vi "CRYResonance Fit.vi"(6 "Y data":dbl=1.0, 7 "Y ref":dbl=1.0, 8 "Algorithm (0)":i32 min=0 max=2 step=1, 11 "Input":cluster{"Freq":dbl, "Magn":dbl}[](array[cluster]) {"Magn" format="%.4f"; "Freq" format="%.2f"}) -> (0 "error":i32, 1 "Q":dbl format="%.2f", 2 "Magn":dbl format="%.2f", 3 "Freq":dbl format="%.2f", 4 "Output":cluster{"FStart":dbl, "Magn":dbl}[](array[cluster]) {"Magn" format="%.2f"; "FStart" format="%.2f"})   [LabVIEW 2013]
uses:
  <vilib>/Analysis/baseanly.llb/A x Vector.vi
  <vilib>/Analysis/7linalg.llb/Solve Linear Equations (single right hand).vi
  <vilib>/Analysis/baseanly.llb/Solve Linear Equations By Cholesky.vi
  <vilib>/Analysis/baseanly.llb/Real Matrix to Compact Array.vi
  <vilib>/Analysis/baseanly.llb/Real Compact Tri-Matrix Linear Eqs.vi
  <vilib>/Analysis/baseanly.llb/Real Inverse Matrix.vi
  <vilib>/Analysis/NI_AALPro.lvlib
  <vilib>/Analysis/NI_AALBase.lvlib
panel:
  out "Magn 2":dbl format="%.2f"
  out "Q 2":dbl format="%.2f"
  out "Freq 2":dbl format="%.2f"
  in  "Y":dbl[](array[numeric])
  out "Matrix A":dbl[][](array[numeric])
  in  "Input 2":cluster{"Freq":dbl, "Magn":dbl}[](array[cluster]) {"Magn" format="%.4f"; "Freq" format="%.2f"}
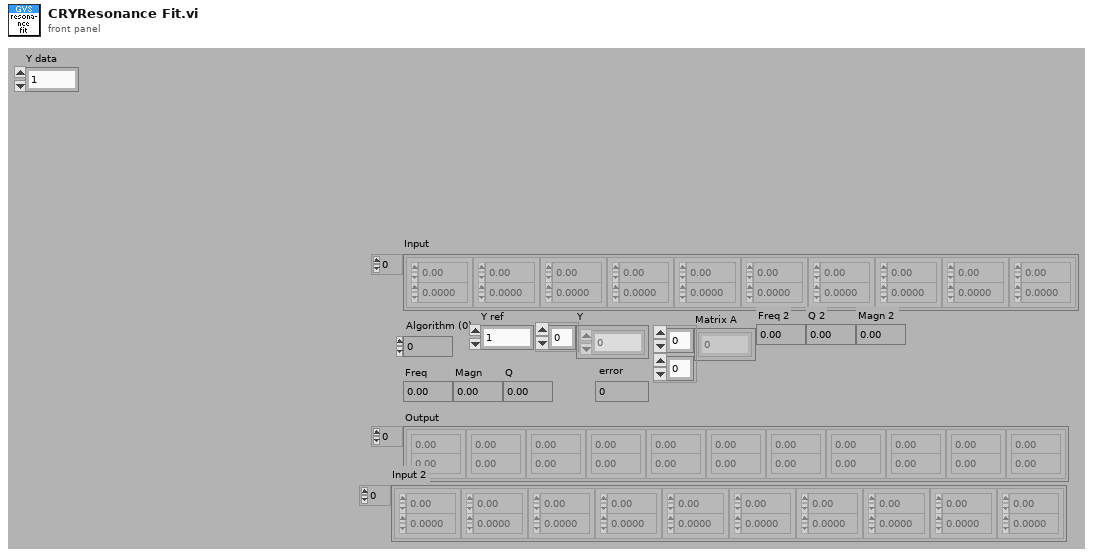
[diagram p1: front panel]
types:
  T1 = typedef "NI_Matrix.lvlib/RealMatrix.ctl" = dbl[][]
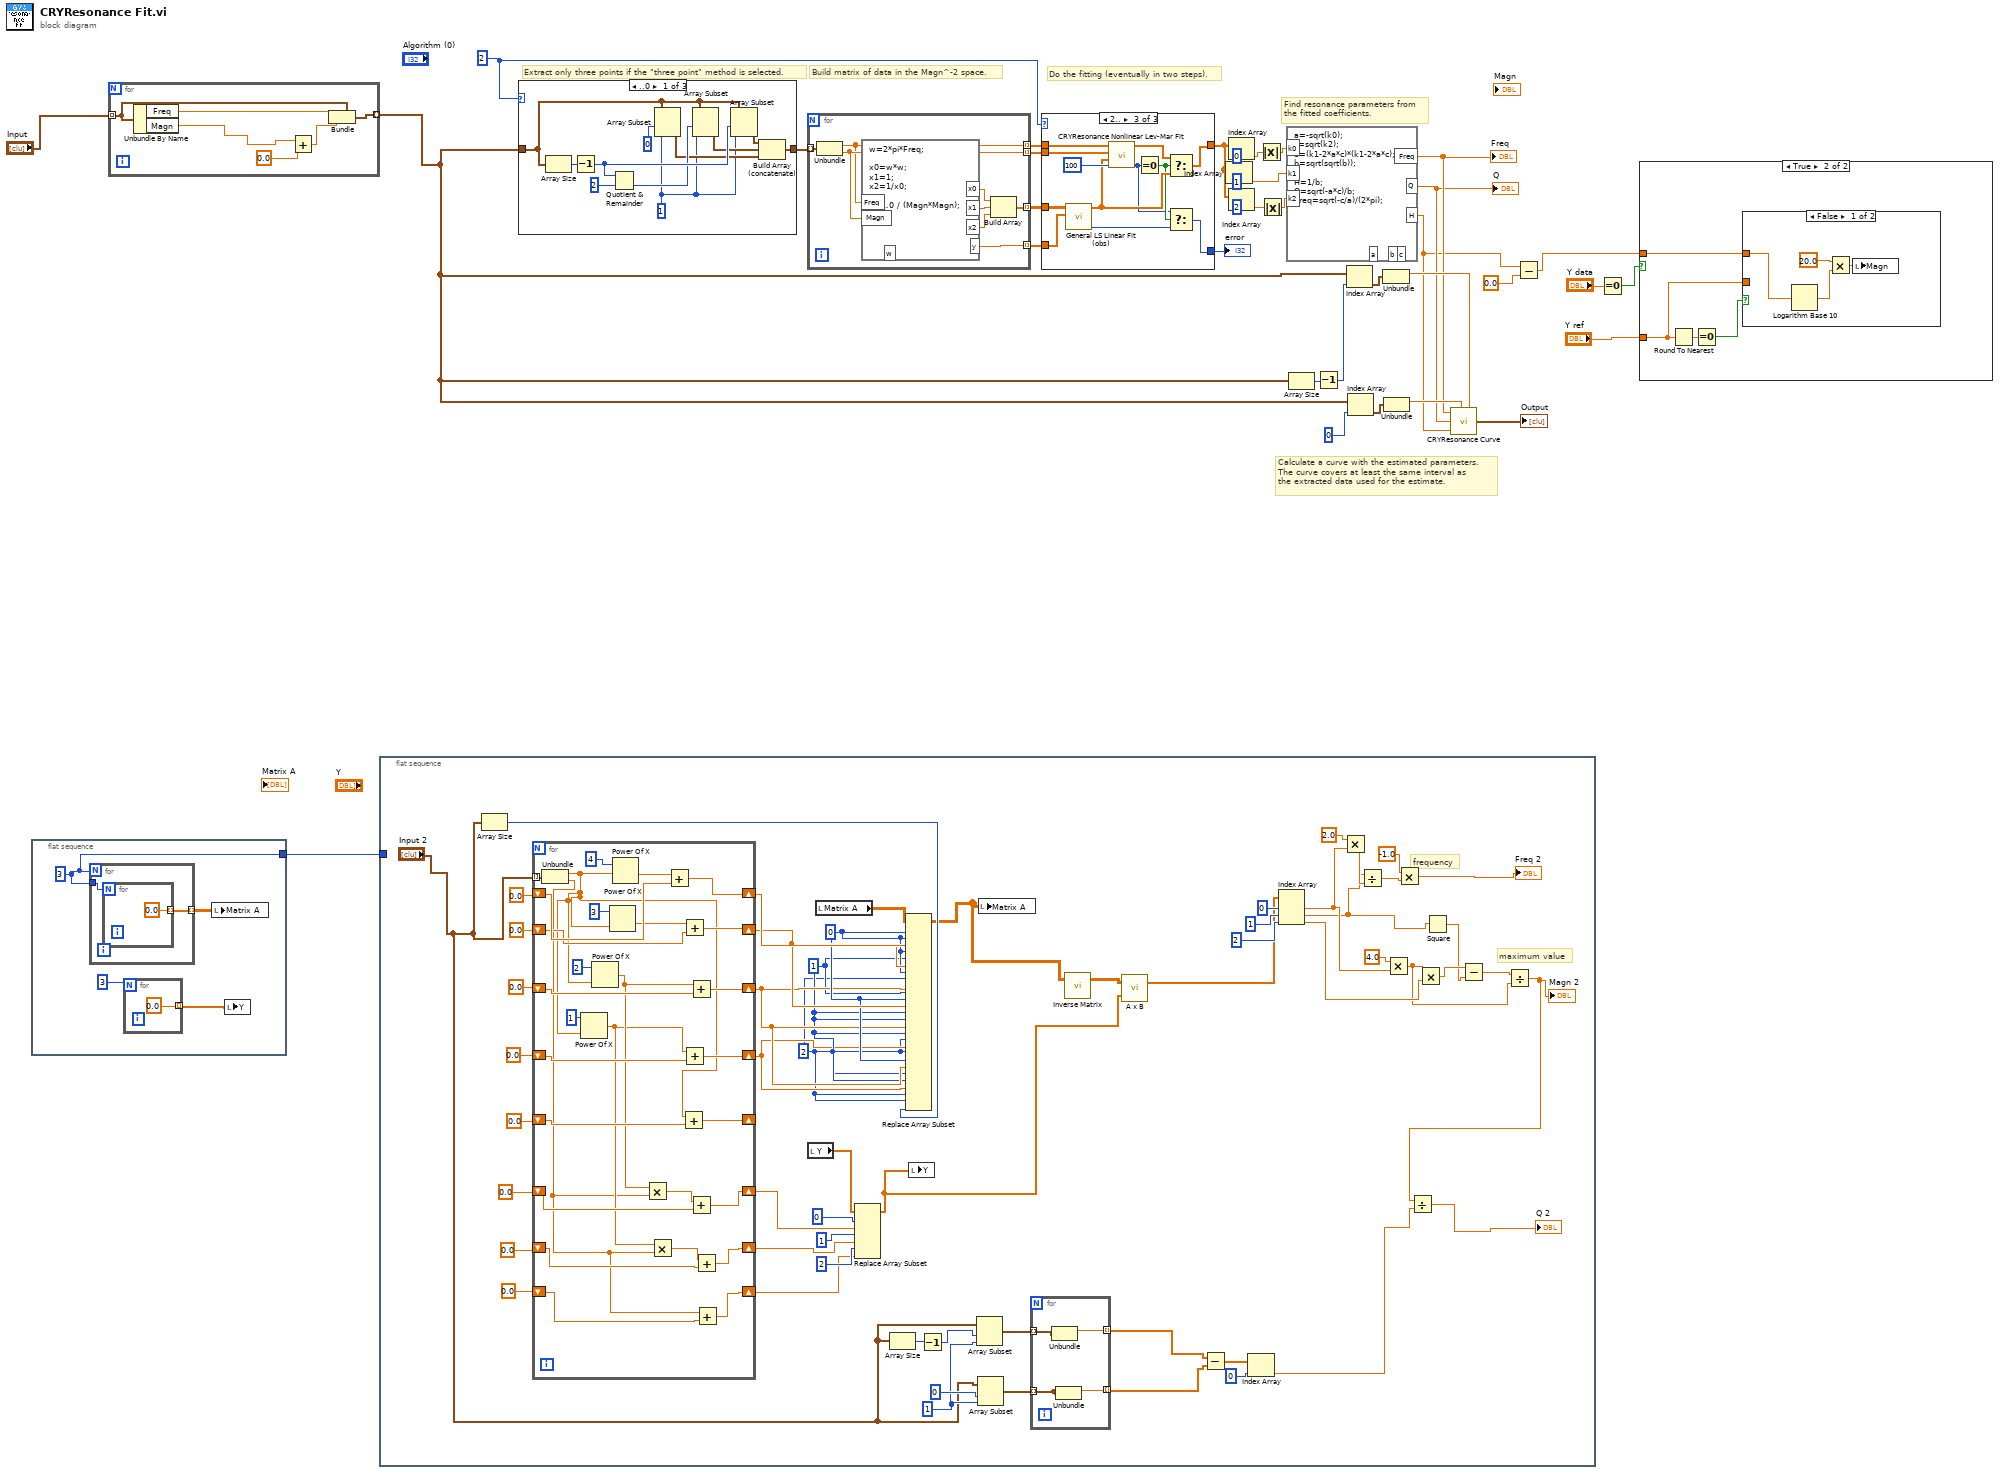
[diagram p0: block diagram]
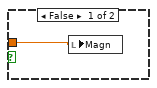
[diagram p2: hidden frame]
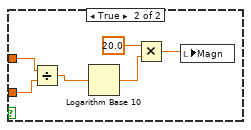
[diagram p3: hidden frame]
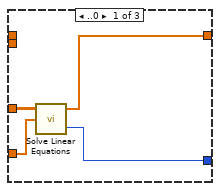
[diagram p4: hidden frame]
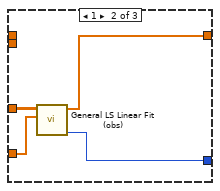
[diagram p5: hidden frame]
diagram:
  w15 = 2
  # "Calculate a curve with the estimated parameters. \nThe curve covers at least the same interval as\nthe extracted data used for the estimate."
  # "Find resonance parameters from\nthe fitted coefficients."
  # "Do the fitting (eventually in two steps)."
  # "Build matrix of data in the Magn^-2 space."
  # "Extract only three points if the \"three point\" method is selected."
  n1 = flat-sequence {
    tunnel: [w36] -> w35
    frame #0 {
      w36 = 3
      n2 = for {
        N: w36 -> [_]
        tunnel: w36 -> [w42]
        tunnel: [w41] -> w39 mode=indexing
        n3 = for {
          N: w42 -> [_]
          tunnel: [0.0] -> w41 mode=indexing
        }
      }
      n4 = for {
        N: 3 -> [_]
        tunnel: [0.0] -> w38 mode=indexing
      }
      n5 = local write "Matrix A"(w39) -> ()
      n6 = local write "Y"(w38) -> ()
    }
  }
  n7 = for {
    tunnel: "Input" -> [w47] mode=indexing
    tunnel: [w48] -> w4 mode=indexing
    n8 = Unbundle By Name(w47) -> ("Freq"=w49:dbl, "Magn"=w44:dbl)
    n9 = Add(x=w44, y=0.0) -> (x+y=w45:dbl)
    n10 = Bundle(cluster=w47, "Freq"=w49, "Magn"=w45) -> (w48:cluster{"Freq":dbl, "Magn":dbl})
  }
  n11 = flat-sequence {
    tunnel: w35 -> [_]
    frame #0 {
      w68 = 1
      w95 = 2
      w97 = 1
      w99 = 0
      # "maximum value"
      # "frequency"
      n12 = Array Size(array="Input 2") -> (size(s)=w58:i32)
      n13 = for {
        tunnel: "Input 2" -> [w140] mode=indexing
        shift-right: [w139] -> w101
        shift-left: 0.0 -> [w138]
        shift-right: [w135] -> w100
        shift-left: 0.0 -> [w134]
        shift-right: [w132] -> w98
        shift-left: 0.0 -> [w131]
        shift-right: [w130] -> w96
        shift-left: 0.0 -> [w129]
        shift-right: [w127] -> _
        shift-left: 0.0 -> [w126]
        shift-right: [w121] -> w89
        shift-left: 0.0 -> [w120]
        shift-right: [w123] -> w87
        shift-left: 0.0 -> [w124]
        shift-right: [w118] -> w85
        shift-left: 0.0 -> [w119]
        n14 = Unbundle(w140) -> ("Freq"=w113:dbl, "Magn"=w112:dbl)
        n15 = Power Of X(1:w113, 2:1) -> (0:w114:dbl)
        n16 = Power Of X(1:w113, 2:2) -> (0:w115:dbl)
        n17 = Power Of X(1:w113, 2:3) -> (0:w116:dbl)
        n18 = Power Of X(1:w113, 2:4) -> (0:w117:dbl)
        n19 = Multiply(x=w115, y=w112) -> (x*y=w122:dbl)
        n20 = Multiply(x=w114, y=w112) -> (x*y=w125:dbl)
        n21 = Add(x=w117, y=w138) -> (x+y=w139:dbl)
        n22 = Add(x=w113, y=w126) -> (x+y=w127:dbl)
        n23 = Add(x=w116, y=w134) -> (x+y=w135:dbl)
        n24 = Add(x=w114, y=w129) -> (x+y=w130:dbl)
        n25 = Add(x=w115, y=w131) -> (x+y=w132:dbl)
        n26 = Add(x=w122, y=w120) -> (x+y=w121:dbl)
        n27 = Add(x=w125, y=w124) -> (x+y=w123:dbl)
        n28 = Add(x=w112, y=w119) -> (x+y=w118:dbl)
      }
      n29 = local read "Y"() -> (w91:dbl[])
      n30 = local read "Matrix A"() -> (w102:dbl[][])
      n31 = Replace Array Subset(array=w91, new element #1=w89, index #1=0, new element #2=w87, index #2=1, new element #3=w85, index #3=2) -> (w55:dbl[])
      n32 = Array Size(array="Input 2") -> (size(s)=w67:i32)
      n33 = Replace Array Subset(array=w102, new element #1=w101, index (row) #1=w99, index (col) #1=w99, new element #2=w100, index (row) #2=w99, index (col) #2=w97, new element #3=w98, index (row) #3=w99, index (col) #3=w95, new element #4=w100, index (row) #4=w97, index (col) #4=w99, new element #5=w98, index (row) #5=w97, index (col) #5=w97, new element #6=w96, index (row) #6=w97, index (col) #6=w95, new element #7=w98, index (row) #7=w95, index (col) #7=w99, new element #8=w96, index (row) #8=w95, index (col) #8=w97, new element #9=w58, index (row) #9=w95, index (col) #9=w95) -> (w57:dbl[][])
      n34 = local write "Y"(w55) -> ()
      n35 = Decrement(x=w67) -> (x-1=w66:i32)
      n36 = Array Subset(array="Input 2", index=w66, length=w68) -> (w65:cluster{"Freq":dbl, "Magn":dbl}[])
      n37 = Array Subset(array="Input 2", index=0, length=w68) -> (w64:cluster{"Freq":dbl, "Magn":dbl}[])
      n38 = local write "Matrix A"(w57) -> ()
      n39 = for {
        tunnel: w65 -> [w111] mode=indexing
        tunnel: [w110] -> w63 mode=indexing
        tunnel: [w109] -> _ mode=indexing
        tunnel: w64 -> [w109] mode=indexing
        tunnel: [w108] -> w62 mode=indexing
        n40 = Unbundle(w111) -> ("Freq"=w110:dbl)  [unwired: 1 out]
        n41 = Unbundle(w109) -> ("Freq"=w108:dbl)  [unwired: 1 out]
      }
      n42 = call-poly <vilib>:"Inverse Matrix.vi"("Input Matrix"=w57) -> ("Inverse Matrix"=w56:T1)  [unwired: 1 in, 1 out]
      n43 = call-poly <vilib>:"A x B.vi"("Vector"=w55, "A"=w56) -> ("A x Vector"=w54:dbl[])  [unwired: 1 out]
      n44 = Subtract(x=w63, y=w62) -> (x-y=w61:dbl[])
      n45 = Index Array(array=w61, index=0) -> (element=w59:dbl)
      n46 = Index Array(array=w54, index #1=0, index #2=1, index #3=2) -> (element #1=w76:dbl, element #2=w74:dbl, element #3=w75:dbl)
      n47 = Multiply(x=2.0, y=w76) -> (x*y=w80:dbl)
      n48 = Divide(x=w74, y=w80) -> (x/y=w79:dbl)
      n49 = Multiply(x=4.0, y=w76) -> (x*y=w70:dbl)
      n50 = Multiply(x=-1.0, y=w79) -> (x*y=→"Freq 2":dbl)
      n51 = Multiply(x=w70, y=w75) -> (x*y=w73:dbl)
      n52 = Square(x=w74) -> (x^2=w72:dbl)
      n53 = Subtract(x=w73, y=w72) -> (x-y=w71:dbl)
      n54 = Divide(x=w71, y=w70) -> (x/y=w50:dbl)
      "Magn 2" <- w50
      n55 = Divide(x=w50, y=w59) -> (x/y=→"Q 2":dbl)
    }
  }
  n56 = case shown="..0" w15 {
    tunnel: w4 -> [w141 w152 w153]
    tunnel: [w142 w152 w153] -> w30
    frame ..0 {
      w143 = 1
      n57 = Array Size(array=w141) -> (size(s)=w150:i32)
      n58 = Decrement(x=w150) -> (x-1=w151:i32)
      n59 = Quotient & Remainder(x=w151, y=2) -> (floor(x/y)=w148:i32)  [unwired: 1 out]
      n60 = Array Subset(array=w141, index=0, length=w143) -> (w147:cluster{"Freq":dbl, "Magn":dbl}[])
      n61 = Array Subset(array=w141, index=w148, length=w143) -> (w146:cluster{"Freq":dbl, "Magn":dbl}[])
      n62 = Array Subset(array=w141, index=w151, length=w143) -> (w145:cluster{"Freq":dbl, "Magn":dbl}[])
      n63 = Build Array (concatenate)(w145, w146, w147) -> (w142:cluster{"Freq":dbl, "Magn":dbl}[])
    }
    frame 1 {
    }
    frame 2.. {
    }
  }
  n64 = for {
    tunnel: w30 -> [w161] mode=indexing
    tunnel: [w158] -> w29 mode=indexing
    tunnel: [w155] -> w28 mode=indexing
    tunnel: [w154] -> w26 mode=indexing
    tunnel: [w160] -> w27 mode=indexing
    n65 = Unbundle(w161) -> ("Freq"=w154:dbl, "Magn"=w160:dbl)
    n66 = formula code="w=2*pi*Freq;\n\nx0=w*w;\nx1=1;\nx2=1/x0;\n\ny=1.0 / (Magn*Magn);"("Freq"=w154, "Magn"=w160) -> ("x0"=w159:dbl, "x1"=w157:dbl, "x2"=w156:dbl, "y"=w155:dbl)  [unwired: 1 out]
    n67 = Build Array(w159, w157, w156) -> (w158:dbl[])
  }
  n68 = case shown="2.." w15 {
    tunnel: w29 -> [w165 w169 w180]
    tunnel: w28 -> [w164 w168 w179]
    tunnel: w27 -> [_ _ w178]
    tunnel: w26 -> [_ _ w177]
    tunnel: [w163 w167 w174] -> w25
    tunnel: [w162 w166 w170] -> w16
    frame ..0 {
      n69 = call-poly <vilib>:"Solve Linear Equations.vi"("Known Vector"=w164, "Input Matrix"=w165) -> ("error"=w162:i32, "Solution Vector"=w163:dbl[])  [unwired: 1 in]
    }
    frame 1 {
      n70 = call <vilib>:"General LS Linear Fit (obs).vi"("H"=w169, "Y"=w168) -> ("Coefficients"=w167:dbl[], "error"=w166:i32)  [unwired: 3 in, 3 out]
    }
    frame 2.. {
      n71 = call <vilib>:"General LS Linear Fit (obs).vi"("H"=w180, "Y"=w179) -> ("Coefficients"=w176:dbl[], "error"=w172:i32)  [unwired: 3 in, 3 out]
      n72 = call "CRYResonance Nonlinear Lev-Mar Fit.vi"("max iteration"=100, "Initial Guess Coefficients"=w176, "Y"=w178, "X"=w177) -> ("error"=w171:i32, "Best Fit Coefficients"=w175:dbl[])  [unwired: 2 in, 3 out]
      n73 = Equal To 0?(x=w171) -> (x = 0?=w173:bool)
      n74 = Select(t=w175, s=w173, f=w176) -> (s? t:f=w174:dbl[])
      n75 = Select(t=w171, s=w173, f=w172) -> (s? t:f=w170:i32)
    }
  }
  "error" <- w16
  n76 = Index Array(array=w25, index=1) -> (element=w31:dbl)
  n77 = Index Array(array=w25, index=0) -> (element=w12:dbl)
  n78 = Index Array(array=w25, index=2) -> (element=w10:dbl)
  n79 = Absolute Value(x=w12) -> (abs(x)=w11:dbl)
  n80 = Absolute Value(x=w10) -> (abs(x)=w9:dbl)
  n81 = formula code="a=-sqrt(k0);\nc=sqrt(k2);\nb=(k1-2*a*c)*(k1-2*a*c);\nb=sqrt(sqrt(b));\n\nH=1/b;\nQ=sqrt(-a*c)/b;\nFreq=sqrt(-c/a)/(2*pi);"("k0"=w11, "k1"=w31, "k2"=w9) -> ("Q"=w13:dbl, "Freq"=w14:dbl, "H"=w2:dbl)  [unwired: 3 out]
  "Freq" <- w14
  "Q" <- w13
  n82 = Array Size(array=w4) -> (size(s)=w23:i32)
  n83 = Decrement(x=w23) -> (x-1=w22:i32)
  n84 = Index Array(array=w4, index=w22) -> (element=w20:cluster{"Freq":dbl, "Magn":dbl})
  n85 = Index Array(array=w4, index=0) -> (element=w19:cluster{"Freq":dbl, "Magn":dbl})
  n86 = Unbundle(w20) -> ("Freq"=w18:dbl)  [unwired: 1 out]
  n87 = Unbundle(w19) -> ("Freq"=w17:dbl)  [unwired: 1 out]
  n88 = call "CRYResonance Curve.vi"("Freq"=w14, "Low Freq"=w17, "Q"=w13, "Magn"=w2, "High Freq"=w18) -> ("Output"=→"Output":cluster{"FStart":dbl, "Magn":dbl}[])  [unwired: 2 in, 2 out]
  n89 = Subtract(x=w2, y=0.0) -> (x-y=w1:dbl)
  n90 = Equal To 0?(x="Y data") -> (x = 0?=w6:bool)
  n91 = case shown="True" w6 {
    tunnel: w1 -> [w182 w184]
    tunnel: "Y ref" -> [_ w183]
    frame False {
      n92 = local write "Magn"(w182) -> ()
    }
    frame True {
      n93 = Round To Nearest(number=w183) -> (nearest integer value=w186:dbl)
      n94 = Equal To 0?(x=w186) -> (x = 0?=w185:bool)
      n95 = case shown="False" w185 {
        tunnel: w184 -> [w187 w196]
        tunnel: w183 -> [_ w195]
        frame False {
          n96 = Logarithm Base 10(1:w187) -> (0:w188:dbl)
          n97 = Multiply(x=20.0, y=w188) -> (x*y=w190:dbl)
          n98 = local write "Magn"(w190) -> ()
        }
        frame True {
          n99 = Divide(x=w196, y=w195) -> (x/y=w192:dbl)
          n100 = Logarithm Base 10(1:w192) -> (0:w193:dbl)
          n101 = Multiply(x=20.0, y=w193) -> (x*y=w191:dbl)
          n102 = local write "Magn"(w191) -> ()
        }
      }
    }
  }
